vi "Get_Cell_Information.vi"(8 "error in (no error)":errorcluster) -> (0 "error out":errorcluster, 3 "Output String":string)   [LabVIEW 2021]
uses:
  Controls/TCP_FGV.ctl
  Controls/Base_Station_Emulator.ctl
  Controls/Cellular_Technology.ctl
  option.ctl
panel:
  in  "option":T1
  in  "Cellular Technology":T2="2G"
  in  "Base Station":T3
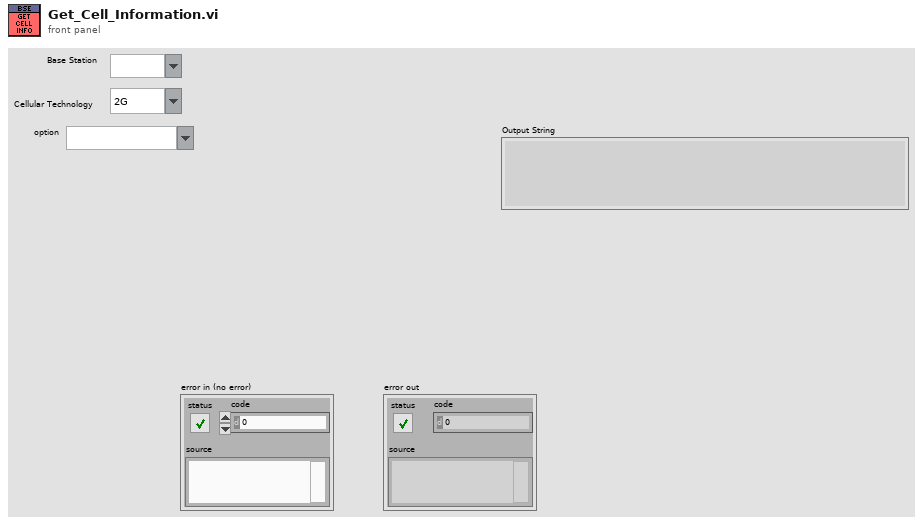
[diagram p1: front panel]
types:
  T1 = typedef "option.ctl" = string
  T2 = typedef "Cellular_Technology.ctl" = string
  T3 = typedef "Base_Station_Emulator.ctl" = string
  T4 = typedef "TCP_FGV.ctl" = enum16{"Open", "Read", "Write", "Close"}
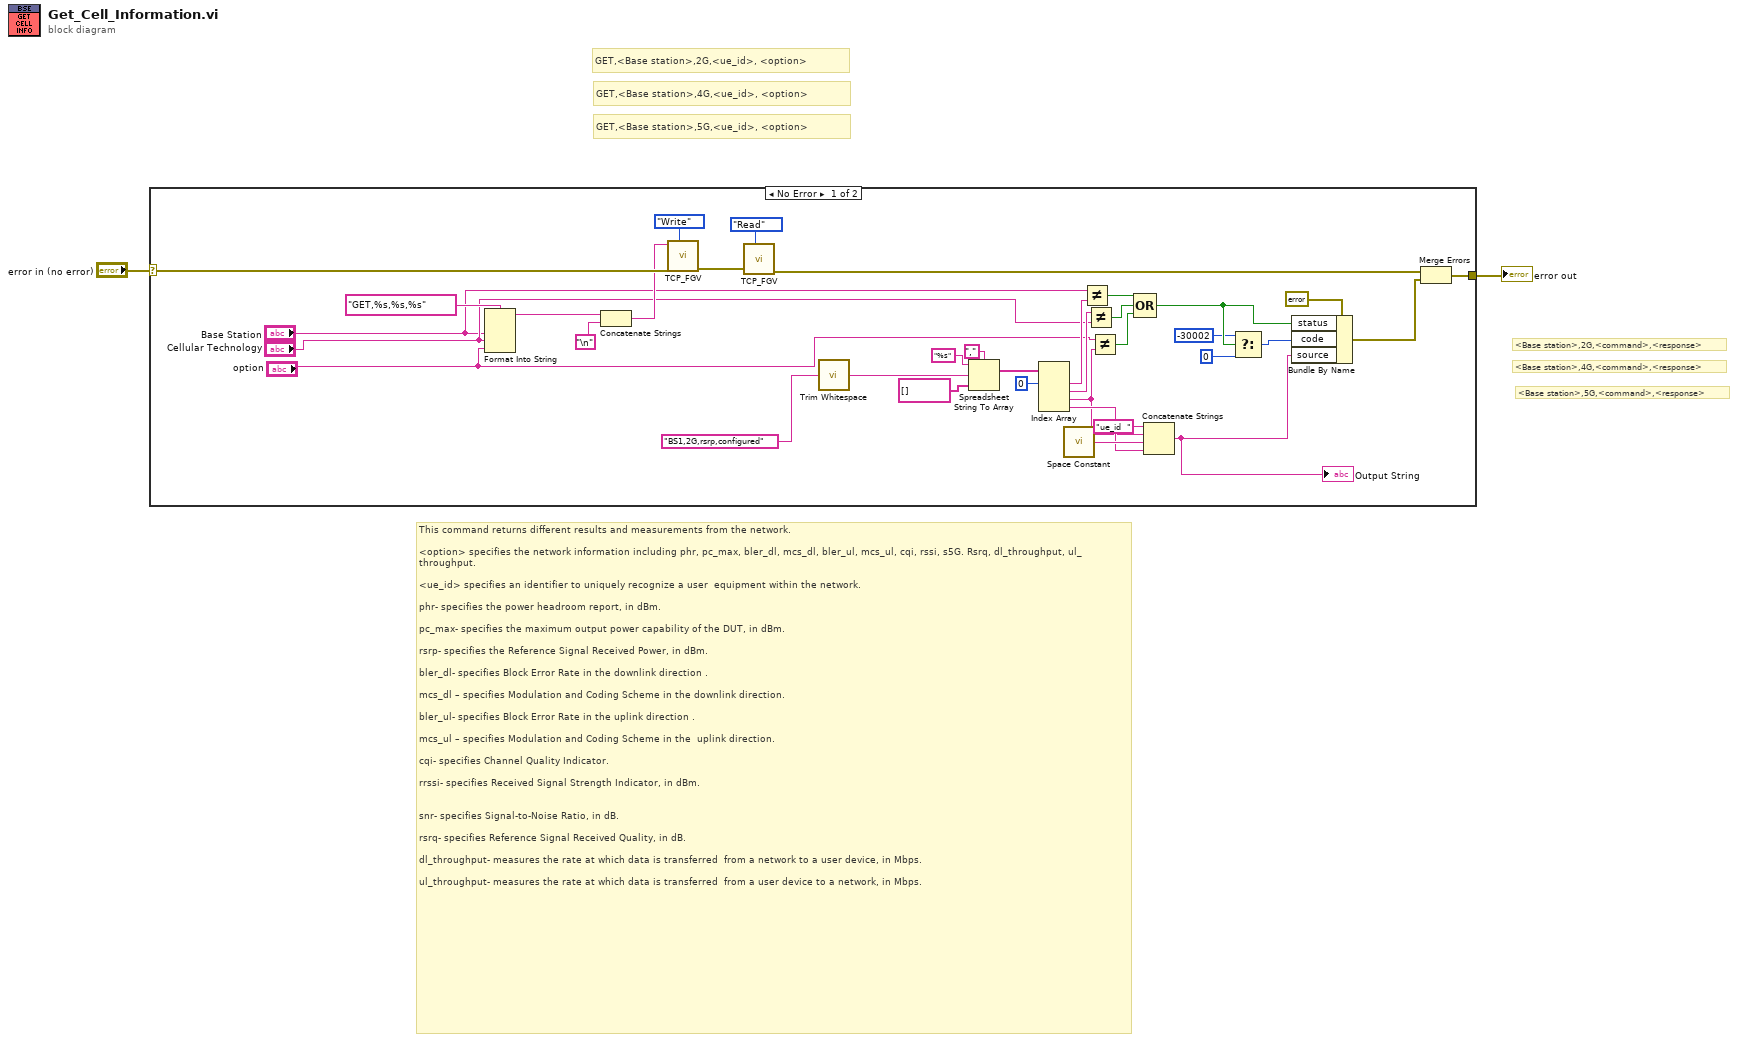
[diagram p0: block diagram]
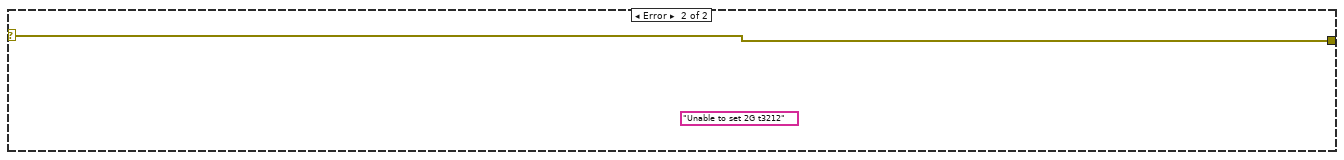
[diagram p2: hidden frame]
diagram:
  # "<Base station>,5G,<command>,<response>"
  # "<Base station>,4G,<command>,<response>"
  # "GET,<Base station>,5G,<ue_id>, <option>"
  # "GET,<Base station>,4G,<ue_id>, <option>"
  # "This command returns different results and measurements from the network.\n\n<option> specifies the network information including phr, pc_max, bler_dl, mcs_dl, bler_ul, mcs_ul, cqi, rssi, s5G. Rsrq, dl_throughput, ul_throughput.  \n\n<ue_id> specifies an identifier to uniquely recognize a user  equipment within the network. \n\nphr- specifies the power headroom report, in dBm. \n\npc_max- specifies the maximum output power capability of the DUT, in dBm. \n\nrsrp- specifies the Reference Signal Received Power, in dBm. \n\nbler_dl- specifies Block Error Rate in the downlink direction . \n\nmcs_dl – specifies Modulation and Coding Scheme in the downlink direction. \n\nbler_ul- specifies Block Error Rate in the uplink direction . \n\nmcs_ul – specifies Modulation and Coding Scheme in the  uplink direction. \n\ncqi- specifies Channel Quality Indicator. \n\nrrssi- specifies Received Signal Strength Indicator, in dBm. \n\n\nsnr- specifies Signal-to-Noise Ratio, in dB. \n\nrsrq- specifies Reference Signal Received Quality, in dB. \n\ndl_throughput- measures the rate at which data is transferred  from a network to a user device, in Mbps. \n\nul_throughput- measures the rate at which data is transferred  from a user device to a network, in Mbps."
  # "GET,<Base station>,2G,<ue_id>, <option>"
  # "<Base station>,2G,<command>,<response>"
  n1 = case shown="No Error" "error in (no error)" {
    selector: "error in (no error)" -> [w37 w39]
    tunnel: [w22 w39] -> w2
    frame No Error {
      n2 = Format Into String(format string="GET,%s,%s,%s", "Base Station", "Cellular Technology", "option") -> (resulting string=w18:string)  [unwired: 2 in, 1 out]
      n3 = Concatenate Strings(w18, "\n") -> (w17:string)
      n4 = call "TCP_FGV.vi"("Command"=w17, "error in (no error)"=w37, "Operation"=TCP_FGV."Write") -> ("error out"=w23:errorcluster)  [unwired: 6 in, 1 out]
      n5 = call "TCP_FGV.vi"("error in (no error)"=w23, "Operation"=TCP_FGV."Read") -> ("error out"=w25:errorcluster)  [unwired: 7 in, 1 out]
      n6 = call <vilib>:"Trim Whitespace.vi"("string"="BS1,2G,rsrp,configured" ("format string")) -> ("trimmed string"=w34:string)  [unwired: 1 in]
      n7 = Spreadsheet String To Array(delimiter (Tab)=",", format string="%s", spreadsheet string=w34, array type (2D Dbl)=string[] []) -> (array=w32:string[])
      n8 = Index Array(array=w32, index #1=0 ("index")) -> (element #1=w14:string, element #2=w33:string, element #3=w4:string, element #4=w8:string)  [unwired: 3 in]
      n9 = call <vilib>:"Space Constant.vi"() -> ("String"=w11:string)
      n10 = Not Equal?(x="Base Station", y=w14) -> (x != y?=w15:bool)
      n11 = Not Equal?(x=w33, y="Cellular Technology") -> (x != y?=w7:bool)
      n12 = Not Equal?(x="option", y=w4) -> (x != y?=w6:bool)
      n13 = Compound Arithmetic op=OR(w15, w7, w6) -> (w35:bool)
      n14 = Concatenate Strings("ue_id  " ("string"), w4, w11, w8) -> (w21:string)
      "Output String" <- w21
      n15 = Select(t=-30002 ("code"), s=w35, f=0 ("code")) -> (s? t:f=w36:i32)
      n16 = Bundle By Name(cluster=errorcluster {"status"=FALSE, "code"=0, "source"=""} ("error constant"), "status"=w35, "code"=w36, "source"=w21) -> (w24:errorcluster)
      n17 = Merge Errors(w25, w24) -> (w22:errorcluster)
    }
    frame Error {
      (unwired) "Unable to set 2G t3212" ("source")
    }
  }
  "error out" <- w2
